vi "CH_LM Action Configuration Save.vi"(0 "Meter Index":i32, 2 "Configuration File Name (\"\")":string, 5 "error in (no error)":errorcluster, 7 "Timeout / ms (3000)":i32=3000, 9 "Lock Timeout / ms (1000)":i32=1000) -> (11 "Lock timed out":bool, 14 "Meter Index":i32, 19 "error out":errorcluster)   [LabVIEW 2012, in "CH_LM.lvlib"]
doc: "This command will store the current configuration to the named configuration file. The named configuration file will be overwritten if the configuration name matches an existing configuration file. \n\n<B>Attention:</B> An attempt to save to the \"Factory Settings\" configuration will raise error 101."
uses:
  CH_LM.lvlib
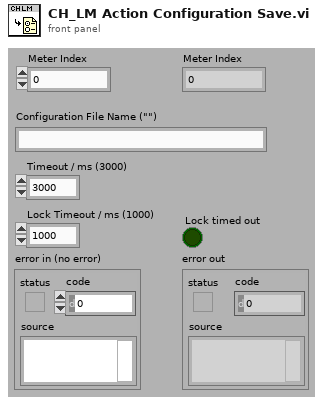
[diagram p1: front panel]
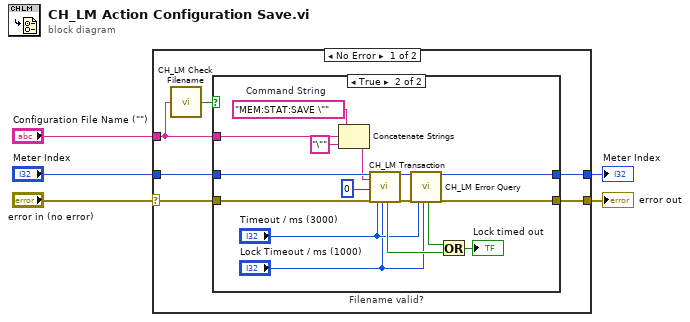
[diagram p0: block diagram]
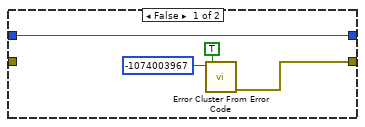
[diagram p2: hidden frame]
diagram:
  n1 = case shown="No Error" "error in (no error)" {
    selector: "error in (no error)" -> [w11 w33]
    tunnel: [w8 w33] -> w5
    tunnel: "Meter Index" -> [w10 w32]
    tunnel: [w9 w32] -> w2
    tunnel: "Configuration File Name (\"\")" -> [w6 _]
    frame No Error {
      n2 = call "CH_LM Check Filename.vi"("Configuration File Name (\"\")"=w6) -> ("Valid"=w7:bool)
      n3 = case "Filename valid?" shown="True" w7 {
        tunnel: w11 -> [_ w31]
        tunnel: w10 -> [w12 w30]
        tunnel: [w12 w26] -> w9
        tunnel: [w13 w25] -> w8
        tunnel: w6 -> [_ w19]
        frame False {
          n4 = call <vilib>:"Error Cluster From Error Code.vi"("show call chain? (False)"=TRUE, "error code (0)"=-1074003967) -> ("error out"=w13:errorcluster)  [unwired: 1 in, 6 out]
        }
        frame True {
          w18 = "MEM:STAT:SAVE \""  # Command String
          n5 = Concatenate Strings(w18, w19, "\"" ("string")) -> (w17:string)
          n6 = call "CH_LM Transaction.vi"("Meter Index"=w30, "Command String"=w17, "NofStrings (-1:all)"=0 ("t"), "error in (no error)"=w31, "Timeout / ms (3000)"="Timeout / ms (3000)", "Lock Timeout / ms (1000)"="Lock Timeout / ms (1000)") -> ("Lock timed out"=w23:bool, "Meter Index"=w28:i32, "error out"=w27:errorcluster)  [unwired: 11 out]
          n7 = call "CH_LM Error Query.vi"("Meter Index"=w28, "error in (no error)"=w27, "Timeout / ms (3000)"="Timeout / ms (3000)", "Lock Timeout / ms (1000)"="Lock Timeout / ms (1000)") -> ("Lock timed out"=w24:bool, "Meter Index"=w26:i32, "error out"=w25:errorcluster)  [unwired: 13 out]
          n8 = Or(x=w24, y=w23) -> (x .or. y?=→"Lock timed out":bool)
        }
      }
    }
    frame Error {
    }
  }
  "error out" <- w5
  "Meter Index" <- w2
